vi "Read Channel info.vi"(8 "error in":errorcluster, 11 "channel in":refnum<class "_Channel.lvclass">) -> (0 "error out":errorcluster, 2 "channel info":T1, 3 "channel out":refnum<class "_Channel.lvclass">)   [LabVIEW 2013, in "_Channel.lvclass"]
uses:
  _Channel.lvclass
  cRIO Repo/ChannelData.ctl
  _Channel.lvclass/_Channel.ctl
  cRIO Repo/_cRIORepo.lvclass
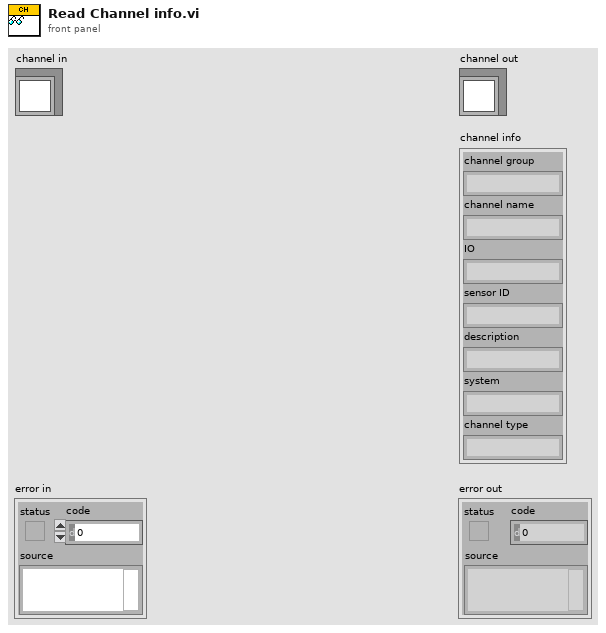
[diagram p1: front panel]
types:
  T1 = typedef "_cRIORepo.lvclass/ChannelData.ctl" = cluster{"channel group":string, "channel name":string, "IO ":string, "sensor ID":string, "description":string, "system":string, "channel type":string}
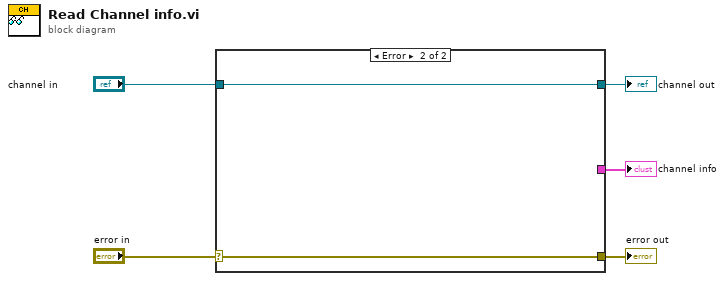
[diagram p0: block diagram]
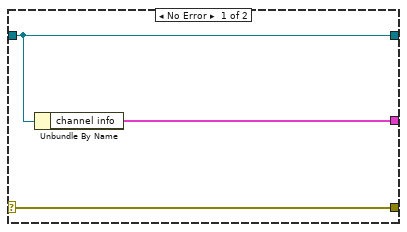
[diagram p2: hidden frame]
diagram:
  n1 = case shown="Error" "error in" {
    selector: "error in" -> [w8 w9]
    tunnel: [w8 w9] -> w4
    tunnel: [w7 w10] -> w2
    tunnel: "channel in" -> [w7 w10]
    tunnel: [w6 _] -> w1
    frame No Error {
      n2 = Unbundle By Name(w7) -> ("channel info"=w6:T1)
    }
    frame Error {
    }
  }
  "error out" <- w4
  "channel out" <- w2
  "channel info" <- w1
